vi "多路CANreset.vi"(8 "错误输入（无错误）":errorcluster, 11 "CAN通道in":u16[](array[numeric])=[81, 82, 83]) -> (0 "错误输出":errorcluster, 3 "CAN 通道out":u16[](array[numeric]))   [LabVIEW 2020]
uses:
  <userlib>/PCANBasic/PCANBasic.lvlib
panel:
  out "function return":u32
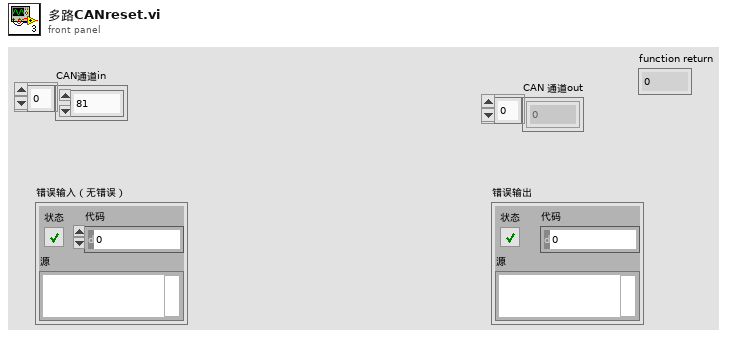
[diagram p1: front panel]
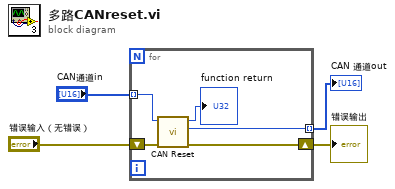
[diagram p0: block diagram]
diagram:
  n1 = for {
    tunnel: "CAN通道in" -> [w9] mode=indexing
    shift-right: [w7] -> w2
    shift-left: "错误输入（无错误）" -> [w8]
    tunnel: [w6] -> w1 mode=indexing
    n2 = call <userlib>:"CAN Reset.vi"("错误输入（无错误）"=w8, "Channel in"=w9) -> ("错误输出"=w7:errorcluster, "Channel out"=w6:u16, "function return"=→"function return":u32)  [unwired: 7 in]
  }
  "CAN 通道out" <- w1
  "错误输出" <- w2
